vi "Window-Position control window.vi"() -> ()   [LabVIEW 2013]
uses:
  Program Files (x86)/National Instruments/LabVIEW 2013/user.lib/My Palettes.lib/Custom Controls/Directional Arrow Buttons/Arrow button-East.ctl
  Program Files (x86)/National Instruments/LabVIEW 2013/user.lib/My Palettes.lib/Custom Controls/Directional Arrow Buttons/Arrow button-West.ctl
  Program Files (x86)/National Instruments/LabVIEW 2013/user.lib/My Palettes.lib/Custom Controls/Directional Arrow Buttons/Arrow button-North.ctl
  Program Files (x86)/National Instruments/LabVIEW 2013/user.lib/My Palettes.lib/Custom Controls/Directional Arrow Buttons/Arrow button-South.ctl
  Program Files (x86)/National Instruments/LabVIEW 2013/user.lib/My Palettes.lib/Custom Controls/Directional Arrow Buttons/Arrow button-North west.ctl
  Program Files (x86)/National Instruments/LabVIEW 2013/user.lib/My Palettes.lib/Custom Controls/Directional Arrow Buttons/Arrow button-North east.ctl
  Program Files (x86)/National Instruments/LabVIEW 2013/user.lib/My Palettes.lib/Custom Controls/Directional Arrow Buttons/Arrow button-South west.ctl
  Program Files (x86)/National Instruments/LabVIEW 2013/user.lib/My Palettes.lib/Custom Controls/Directional Arrow Buttons/Arrow button-South east.ctl
  User Interface/Windows/Position control window/Typedefs/Pos Ctrl States.ctl
  User Interface/Windows/Position control window/Typedefs/Pos Ctrl queue data cluster.ctl
  User Interface/Windows/Position control window/Typedefs/Pos Ctrl window refs cluster.ctl
  Typedefs/Movement mode.ctl
  Peripherals Control/XYZ Stage/Typedefs/XYZ stage states.ctl
  Typedefs/Axis of movement.ctl
  User Interface/Windows/Position control window/Globals/Pos ctrl window globals.vi
  Global Variables/General Globals.vi
  Peripherals Control/XYZ Stage/Globals/gl_XYZStage globals.vi
  Typedefs/Save-Load enum.ctl
  Peripherals Control/XYZ Stage/Typedefs/XYZ channel ring.ctl
  Peripherals Control/XYZ Stage/Typedefs/XYZ stage data.ctl
panel:
  in  "Motor E-Stop":bool
  out "# elements in queue":i32
  out "x+1":dbl
  in  "Y Coordinate ctrl":sgl min=-20000 max=20000 step=0.1 format="Y:%#_g um"
  out "Close":bool
  in  "Z step (um)":sgl=1.0 min=0.1 max=1000 step=0.1 format="%#_6f"
  in  "Z Coordinate ctrl":sgl min=-20000 max=20000 step=0.1 format="Z:%#.1f um"
  in  "Z move down":T1
  in  "Z move up":T2
  out "Z-axis section":string
  in  "Step = size of image":bool
  in  "XY step (um)":sgl=1.0 min=0.1 max=10000 step=0.1
  out "State":T3
  out "Last button name":string
  out "Event loop":i32
  out "Elapsed Time (s)":dbl format="%#.1g"
  in  "Speed setting ctrl":i32=1000 min=1000 max=50000 step=1 format="Speed\n%#_6g\num/sec"
  in  "Speed down":bool
  in  "Speed up":bool
  in  "X Coordinate ctrl":sgl min=-20000 max=20000 step=0.1 format="X:%#_g um"
  in  "Down-right":T4
  in  "Down-left":T5
  in  "Up-right":T6
  in  "Up-left":T7
  in  "Down":T1
  in  "Up":T2
  in  "Left":T8
  in  "Right":T9
  # "Speed"
  # "X-Y Movement"
  # "Z Movement"
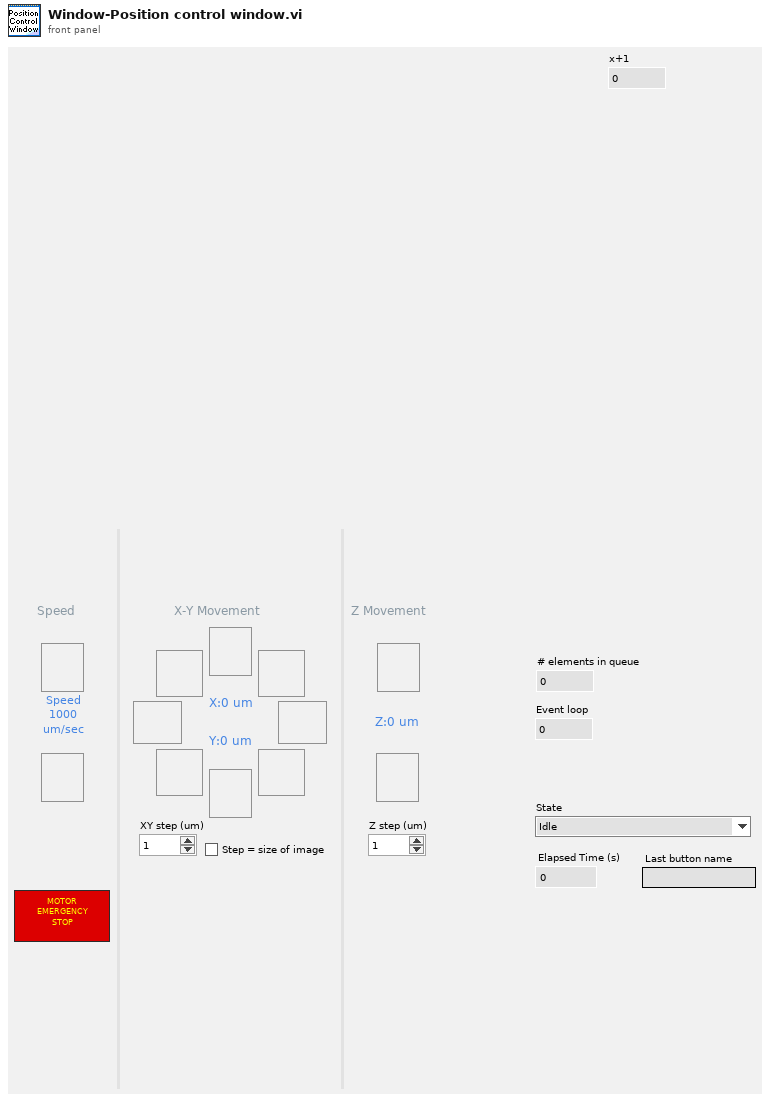
[diagram p1: front panel]
types:
  T1 = typedef "Arrow button-South.ctl" = bool
  T2 = typedef "Arrow button-North.ctl" = bool
  T3 = typedef "Pos Ctrl States.ctl" = enum16{"Idle", "Count-down", "Request single step (ack.)", "Request single step (no ack.)", "Request continuous movement", "Request movement stop"}
  T4 = typedef "Arrow button-South east.ctl" = bool
  T5 = typedef "Arrow button-South west.ctl" = bool
  T6 = typedef "Arrow button-North east.ctl" = bool
  T7 = typedef "Arrow button-North west.ctl" = bool
  T8 = typedef "Arrow button-West.ctl" = bool
  T9 = typedef "Arrow button-East.ctl" = bool
  T10 = typedef "Pos Ctrl window refs cluster.ctl" = cluster{"menu reference":refnum<k9>, "X Coordinate ctrl":refnum<vi>, "Y Coordinate ctrl":refnum<vi>, "Z Coordinate ctrl":refnum<vi>, "Speed setting ctrl":refnum<vi>, "Up":refnum<vi>, "Down":refnum<vi>, "Left":refnum<vi>, "Right":refnum<vi>, "Z move up":refnum<vi>, "Z move down":refnum<vi>, "Down-left":refnum<vi>, "Down-right":refnum<vi>, "Up-left":refnum<vi>, "Up-right":refnum<vi>, "Step = size of image":refnum<vi>, "XY step (um)":refnum<vi>, "Z step (um)":refnum<vi>}
  T11 = typedef "Pos Ctrl queue data cluster.ctl" = cluster{"State":T3, "variant":variant}
  T12 = enum32{"Invalid", "Standard", "Closed", "Hidden", "Minimized", "Maximized"}
  T13 = typedef "XYZ stage states.ctl" = enum16{"Dequeue", "Initialize", "Read Position", "Read Speed Setting", "Move", "Set Max Speed", "Reset Axis", "Stop all movement"}
  T14 = typedef "Axis of movement.ctl" = enum16{"None", "X-axis", "Y-Axis", "-45 deg Axis", "+45 deg Axis", "Z-Axis"}
  T15 = enum8{"Enabled", "Disabled", "Disabled and Grayed Out"}
  T16 = typedef "XYZ stage data.ctl" = cluster{"Command":T13, "Channel":T17, "X":sgl, "Y":sgl, "Z":sgl, "Speed":i32, "Zero":bool, "Use acknowledgement?":bool}
  T17 = typedef "XYZ channel ring.ctl" = string
  T18 = typedef "Save-Load enum.ctl" = enum16{"Save to file", "Load from file", "Compare from file"}
  T19 = typedef "Movement mode.ctl" = enum16{"Move the frame", "Move the feature"}
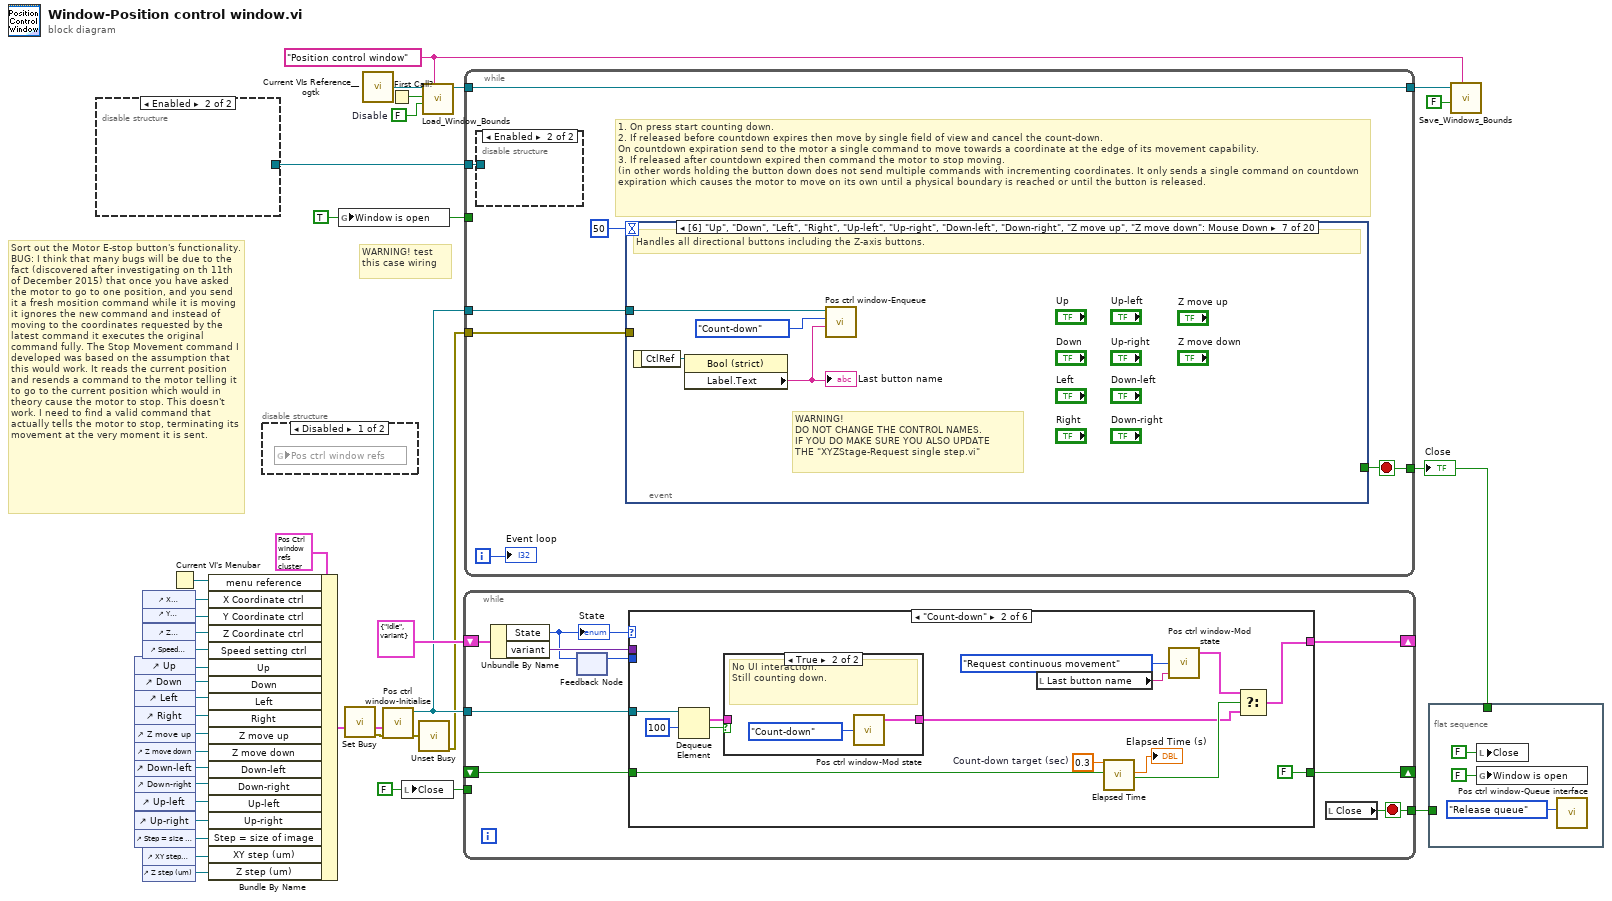
[diagram p0: block diagram]
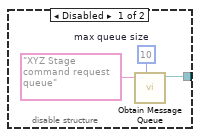
[diagram p2: hidden frame]
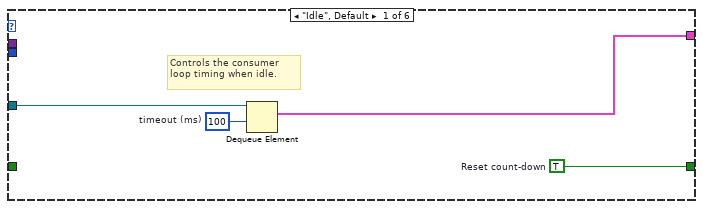
[diagram p4: hidden frame]
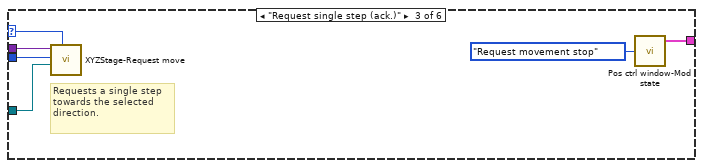
[diagram p6: hidden frame]
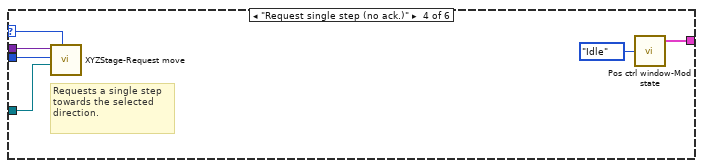
[diagram p7: hidden frame]
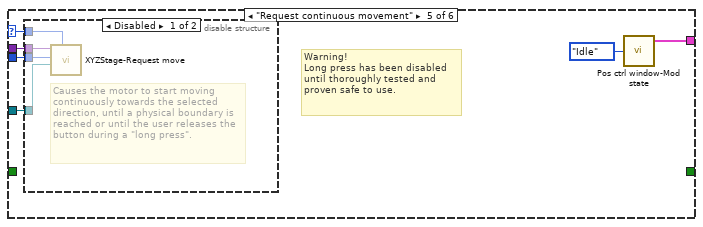
[diagram p8: hidden frame]
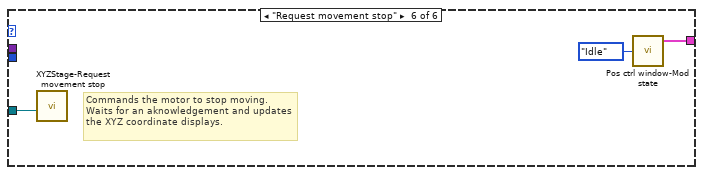
[diagram p10: hidden frame]
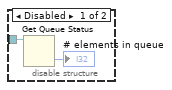
[diagram p11: hidden frame]
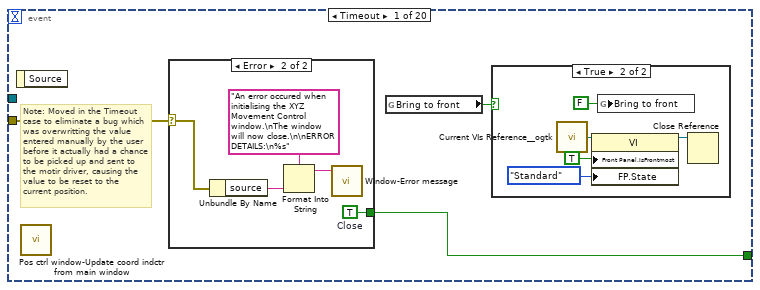
[diagram p12: hidden frame]
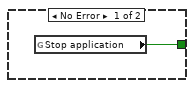
[diagram p14: hidden frame]
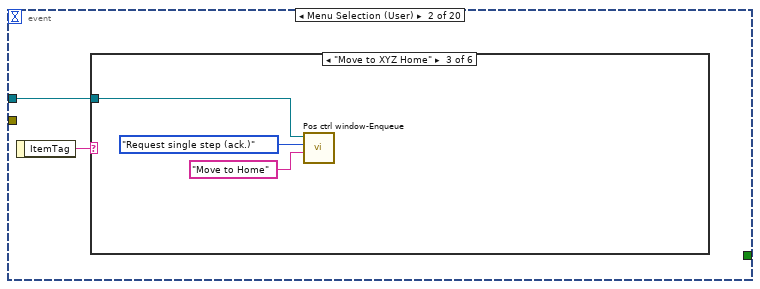
[diagram p15: hidden frame]
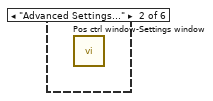
[diagram p17: hidden frame]
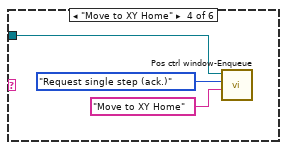
[diagram p18: hidden frame]
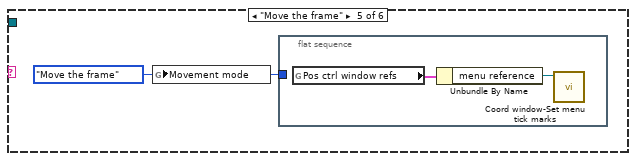
[diagram p19: hidden frame]
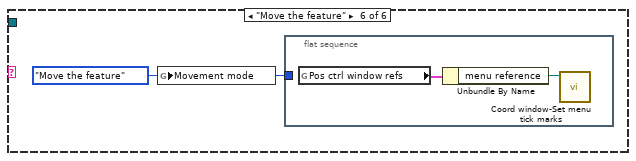
[diagram p20: hidden frame]
diagram:
  w10 = FALSE  # Disable
  w8 = "Position control window" ("Window Name (i.e. Key)")
  w14 = TRUE ("Bring to front")
  w25 = FALSE ("Close")
  # "Sort out the Motor E-stop button's functionality.\nBUG: I think that many bugs will be due to the fact (discovered after investigating on th 11th of December 2015) that once you have asked the motor to go to one position, and you send it a fresh mosition command while it is moving it ignores the new command and instead of moving to the coordinates requested by the latest command it executes the original command fully. The Stop Movement command I developed was based on the assumption that this would work. It reads the current position and resends a command to the motor telling it to go to the current position which would in theory cause the motor to stop. This doesn't work. I need to find a valid command that actually tells the motor to stop, terminating its movement at the very moment it is sent."
  # "WARNING! test this case wiring"
  n1 = disable-structure shown="Enabled" {
    disable-tunnel: [w38 _] -> w6
    frame Disabled {
      w40 = 10  # max queue size
      n2 = call "Obtain Message Queue.vi"("max queue size (-1, unlimited)"=w40, "Queue name"="XYZ Stage command request queue") -> ("Message Queue"=w38:refnum<queue>)  [unwired: 8 in, 1 out]
    }
    frame Enabled {
    }
  }
  n3 = control-ref of="Up"() -> (w35:refnum<vi>)
  n4 = control-ref of="Down"() -> (w34:refnum<vi>)
  n5 = control-ref of="Left"() -> (w33:refnum<vi>)
  n6 = control-ref of="Right"() -> (w32:refnum<vi>)
  n7 = control-ref of="Z move up"() -> (w31:refnum<vi>)
  n8 = control-ref of="Z move down"() -> (w30:refnum<vi>)
  n9 = control-ref of="Down-left"() -> (w29:refnum<vi>)
  n10 = control-ref of="Down-right"() -> (w28:refnum<vi>)
  n11 = control-ref of="Up-left"() -> (w27:refnum<vi>)
  n12 = control-ref of="Up-right"() -> (w26:refnum<vi>)
  n13 = control-ref of="Step = size of image"() -> (w23:refnum<vi>)
  n14 = control-ref of="X Coordinate ctrl"() -> (w18:refnum<vi>)
  n15 = control-ref of="Y Coordinate ctrl"() -> (w17:refnum<vi>)
  n16 = control-ref of="Z Coordinate ctrl"() -> (w16:refnum<vi>)
  n17 = control-ref of="Speed setting ctrl"() -> (w15:refnum<vi>)
  n18 = control-ref of="XY step (um)"() -> (w22:refnum<vi>)
  n19 = control-ref of="Z step (um)"() -> (w21:refnum<vi>)
  n20 = Current VI's Menubar() -> (w5:refnum<k9>)
  n21 = Bundle By Name(cluster=T10 {"menu reference"=refnum, "X Coordinate ctrl"=refnum, "Y Coordinate ctrl"=refnum, "Z Coordinate ctrl"=refnum, "Speed setting ctrl"=refnum, "Up"=refnum, "Down"=refnum, "Left"=refnum, "Right"=refnum, "Z move up"=refnum, "Z move down"=refnum, "Down-left"=refnum, "Down-right"=refnum, "Up-left"=refnum, "Up-right"=refnum, "Step = size of image"=refnum, "XY step (um)"=refnum, "Z step (um)"=refnum} ("Pos ctrl window refs"), "menu reference"=w5, "X Coordinate ctrl"=w18, "Y Coordinate ctrl"=w17, "Z Coordinate ctrl"=w16, "Speed setting ctrl"=w15, "Up"=w35, "Down"=w34, "Left"=w33, "Right"=w32, "Z move up"=w31, "Z move down"=w30, "Down-left"=w29, "Down-right"=w28, "Up-left"=w27, "Up-right"=w26, "Step = size of image"=w23, "XY step (um)"=w22, "Z step (um)"=w21) -> (w19:T10)
  n22 = disable-structure shown="Disabled" {
    frame Disabled {
      n23 = global read "Pos ctrl window globals.vi" "Pos ctrl window refs"() -> ()  [unwired: 1 in]
    }
    frame Enabled {
    }
  }
  n24 = global write "Pos ctrl window globals.vi" "Window is open"(w14) -> ()
  n25 = call <vilib>:"Set Busy.vi"() -> ("error out"=w3:errorcluster)  [unwired: 10 in, 1 out]
  n26 = call "Current VIs Reference__ogtk.vi"() -> ("Current VI's reference"=w13:refnum<vi>)  [unwired: 5 in]
  n27 = call "Pos ctrl window-Initialise.vi"("error in (no error)"=w3, "Pos ctrl window refs"=w19) -> ("error out"=w2:errorcluster, "XYZ movement ctrl window queue ref"=w20:refnum<queue>)  [unwired: 8 in]
  n28 = First Call?() -> (First Call?: T/F=w11:bool)
  n29 = local write "Close"(w25) -> ()
  n30 = call <vilib>:"Unset Busy.vi"("error in (no error)"=w2) -> ("error out"=w1:errorcluster)  [unwired: 10 in]
  n31 = call "Load_Window_Bounds.vi"("Window Name (i.e. Key)"=w8, "Disable"=w10, "First Call"=w11, "Window VI's Ref"=w13) -> ("reference out"=w12:refnum<vi>)  [unwired: 4 in, 3 out]
  n32 = while {
    tunnel: w20 -> [w49]
    shift-right: [w48] -> _
    shift-left: T11 {"State"=enum."Idle", "variant"=variant} ("Pos Ctrl queue data cluster") -> [w45]
    shift-right: [w47] -> _
    shift-left: _ -> [w46]
    tunnel: w25 -> [_]
    tunnel: [w41] -> w24
    stop <- w41 stop-if-true
    n33 = Unbundle By Name(w45) -> ("State"=w43:T3, "variant"=w44:variant)
    "State" <- w43
    n34 = feedback-in #1(w43) -> ()
    n35 = feedback #1() -> (w42:T3)  [unwired: 1 in]
    n36 = case shown="\"Count-down\"" w43 {
      selector: w43 -> [_ _ w71 w77 w83 _]
      tunnel: w49 -> [w52 w66 w73 w79 w86 w93]
      tunnel: [w50 w55 w75 w81 w87 w94] -> w48
      tunnel: [w51 FALSE _ _ _ _] -> w47
      tunnel: w46 -> [_ w63 _ _ _ _]
      tunnel: w44 -> [_ _ w74 w80 w85 _]
      tunnel: w42 -> [_ _ w72 w78 w84 _]
      frame "Idle", Default {
        w51 = TRUE  # Reset count-down
        w53 = 100  # timeout (ms)
        # "Controls the consumer loop timing when idle."
        n37 = Dequeue Element(queue=w52, timeout in ms (-1)=w53) -> (element=w50:T11)  [unwired: 1 in, 3 out]
      }
      frame "Count-down" {
        w64 = 0.3  # Count-down target (sec)
        n38 = Dequeue Element(queue=w66, timeout in ms (-1)=100) -> (element=w61:T11, timed out?=w62:bool)  [unwired: 1 in, 2 out]
        n39 = case shown="True" w62 {
          tunnel: [w68 w69] -> w56
          tunnel: w61 -> [w68 _]
          frame False {
            # "Queue element received.\nUI interaction detected."
          }
          frame True {
            # "No UI interaction.\nStill counting down."
            n40 = call "Pos ctrl window-Mod state.vi"("States"=Pos_Ctrl_States."Count-down") -> ("Modified queue element"=w69:T11)  [unwired: 4 in]
          }
        }
        n41 = local read "Last button name"() -> (w54:string)
        n42 = call "Elapsed Time"("Time Target (s)"=w64, "Reset"=w63) -> ("Elapsed Time (s)"=→"Elapsed Time (s)":dbl, "Time has Elapsed"=w57:bool)  [unwired: 10 in, 6 out]
        n43 = call "Pos ctrl window-Mod state.vi"("variant"=w54, "States"=Pos_Ctrl_States."Request continuous movement") -> ("Modified queue element"=w59:T11)  [unwired: 3 in]
        n44 = Select(t=w59, s=w57, f=w56) -> (s? t:f=w55:T11)
      }
      frame "Request single step (ack.)" {
        # "Requests a single step towards the selected direction."
        n45 = call "XYZStage-Request move.vi"("Current State"=w71, "Pos ctrl window queue"=w73, "Previous State"=w72, "variant"=w74) -> ()  [unwired: 8 in]
        n46 = call "Pos ctrl window-Mod state.vi"("States"=Pos_Ctrl_States."Request movement stop") -> ("Modified queue element"=w75:T11)  [unwired: 4 in]
      }
      frame "Request single step (no ack.)" {
        # "Requests a single step towards the selected direction."
        n47 = call "XYZStage-Request move.vi"("Current State"=w77, "Pos ctrl window queue"=w79, "Previous State"=w78, "variant"=w80) -> ()  [unwired: 8 in]
        n48 = call "Pos ctrl window-Mod state.vi"("States"=Pos_Ctrl_States."Idle") -> ("Modified queue element"=w81:T11)  [unwired: 4 in]
      }
      frame "Request continuous movement" {
        # "Warning!\nLong press has been disabled until thoroughly tested and proven safe to use."
        n49 = disable-structure shown="Disabled" {
          disable-tunnel: w86 -> [w92 _]
          disable-tunnel: w85 -> [w91 _]
          disable-tunnel: w84 -> [w90 _]
          disable-tunnel: w83 -> [w89 _]
          frame Disabled {
            # "Causes the motor to start moving continuously towards the selected direction, until a physical boundary is reached or until the user releases the button during a \"long press\"."
            n50 = call "XYZStage-Request move.vi"("Current State"=w89, "Pos ctrl window queue"=w92, "Previous State"=w90, "variant"=w91) -> ()  [unwired: 8 in]
          }
          frame Enabled {
          }
        }
        n51 = call "Pos ctrl window-Mod state.vi"("States"=Pos_Ctrl_States."Idle") -> ("Modified queue element"=w87:T11)  [unwired: 4 in]
      }
      frame "Request movement stop" {
        # "Commands the motor to stop moving.\nWaits for an aknowledgement and updates the XYZ coordinate displays."
        n52 = call "XYZStage-Request movement stop.vi"("Pos ctrl window queue"=w93) -> ()  [unwired: 11 in]
        n53 = call "Pos ctrl window-Mod state.vi"("States"=Pos_Ctrl_States."Idle") -> ("Modified queue element"=w94:T11)  [unwired: 4 in]
      }
    }
    n54 = local read "Close"() -> (w41:bool)
  }
  n55 = while {
    tunnel: w20 -> [w101]
    tunnel: [w99] -> w4
    tunnel: w1 -> [w98]
    tunnel: w14 -> [_]
    tunnel: w12 -> [w97]
    tunnel: [w97] -> w9
    tunnel: w6 -> [w96]
    i -> [w100]
    stop <- w99 stop-if-true
    # "1. On press start counting down.\n2. If released before countdown expires then move by single field of view and cancel the count-down.\nOn countdown expiration send to the motor a single command to move towards a coordinate at the edge of its movement capability.\n3. If released after countdown expired then command the motor to stop moving.\n(in other words holding the button down does not send multiple commands with incrementing coordinates. It only sends a single command on countdown expiration which causes the motor to move on its own until a physical boundary is reached or until the button is released."
    n56 = disable-structure shown="Enabled" {
      disable-tunnel: w96 -> [w104 _]
      frame Disabled {
        n57 = Get Queue Status(queue=w104) -> (# elements in queue=→"# elements in queue":i32)  [unwired: 2 in, 7 out]
      }
      frame Enabled {
      }
    }
    n58 = event shown="[6] \"Up\", \"Down\", \"Left\", \"Right\", \"Up-left\", \"Up-right\", \"Down-left\", \"Down-right\", \"Z move up\", \"Z move down\": Mouse Down" {
      selector: _ -> [_ _ _ _ _ _ _ _ _ _ _ _ _ _ _ _ _ _ _ _]
      dyn-events: _ -> [_ _ _ _ _ _ _ _ _ _ _ _ _ _ _ _ _ _ _ _]
      timeout: 50 -> [_ _ _ _ _ _ _ _ _ _ _ _ _ _ _ _ _ _ _ _]
      tunnel: w101 -> [_ w119 w136 _ _ _ w172 w175 w183 _ _ _ _ _ _ _ _ _ w199 _]
      tunnel: [w106 _ _ _ _ _ _ _ _ _ _ _ _ _ _ _ _ _ _ TRUE] -> w99
      tunnel: w98 -> [w107 _ _ _ _ _ _ _ _ _ _ _ _ _ _ _ _ _ _ _]
      event Timeout {
        # "Note: Moved in the Timeout case to eliminate a bug which was overwritting the value entered manually by the user before it actually had a chance to be picked up and sent to the motir driver, causing the value to be reset to the current position."
        n59 = event-data() -> ()  [unwired: 1 in, 1 out]
        n60 = call "Pos ctrl window-Update coord indctr from main window.vi"() -> ()  [unwired: 12 in]
        n61 = case shown="Error" w107 {
          selector: w107 -> [_ w115]
          tunnel: [w113 w118] -> w106
          frame No Error {
            n62 = global read "General Globals.vi" "Stop application"() -> (w113:bool)
          }
          frame Error {
            w118 = TRUE  # Close
            n63 = Unbundle By Name(w115) -> ("source"=w114:string)
            n64 = Format Into String(format string="An error occured when initialising the XYZ Movement Control window.\nThe window will now close.\n\nERROR DETAILS:\n%s" ("Error Source"), w114) -> (resulting string=w117:string)  [unwired: 2 in, 1 out]
            n65 = call "Window-Error message.vi"("Message"=w117) -> ()  [unwired: 10 in, 1 out]
          }
        }
        n66 = global read "Pos ctrl window globals.vi" "Bring to front"() -> (w105:bool)
        n67 = case shown="True" w105 {
          frame False {
          }
          frame True {
            n68 = call "Current VIs Reference__ogtk.vi"() -> ("Current VI's reference"=w111:refnum<vi>)  [unwired: 5 in]
            n69 = property class="VI"(reference=w111, "Front Panel.IsFrontmost"=TRUE ("Front Panel Window:Is Frontmost"), "FP.State"=T12."Standard" ("Front Panel Window:State")) -> (reference out=w110:refnum<vi>)  [unwired: 1 in, 1 out]
            n70 = global write "Pos ctrl window globals.vi" "Bring to front"(FALSE ("Bring to front")) -> ()
            n71 = Close Reference(reference=w110) -> ()  [unwired: 1 in, 1 out]
          }
        }
      }
      event Menu Selection (User) {
        n72 = event-data() -> ("ItemTag"=w120:string)  [unwired: 1 in]
        n73 = case shown="\"Move to XYZ Home\"" w120 {
          tunnel: w119 -> [_ _ w121 w124 _ _]
          frame Default {
          }
          frame "Advanced Settings..." {
            n74 = call "Pos ctrl window-Settings window.vi"() -> ()  [unwired: 11 in, 1 out]
          }
          frame "Move to XYZ Home" {
            n75 = call "Pos ctrl window-Enqueue.vi"("variant"="Move to Home" ("Last button name"), "States"=Pos_Ctrl_States."Request single step (ack.)", "Pos ctrl window queue"=w121) -> ()  [unwired: 8 in, 1 out]
          }
          frame "Move to XY Home" {
            n76 = call "Pos ctrl window-Enqueue.vi"("variant"="Move to XY Home" ("Last button name"), "States"=Pos_Ctrl_States."Request single step (ack.)", "Pos ctrl window queue"=w124) -> ()  [unwired: 8 in, 1 out]
          }
          frame "Move the frame" {
            w127 = Movement_mode."Move the frame" ("Movement mode")
            n77 = global write "Pos ctrl window globals.vi" "Movement mode"(w127) -> ()
            n78 = flat-sequence {
              tunnel: w127 -> [_]
              frame #0 {
                n79 = global read "Pos ctrl window globals.vi" "Pos ctrl window refs"() -> (w128:T10)
                n80 = Unbundle By Name(w128) -> ("menu reference"=w129:refnum<k9>)
                n81 = call "Coord window-Set menu tick marks.vi"("Menu in"=w129) -> ()  [unwired: 9 in, 2 out]
              }
            }
          }
          frame "Move the feature" {
            w130 = Movement_mode."Move the feature" ("Movement mode")
            n82 = global write "Pos ctrl window globals.vi" "Movement mode"(w130) -> ()
            n83 = flat-sequence {
              tunnel: w130 -> [_]
              frame #0 {
                n84 = global read "Pos ctrl window globals.vi" "Pos ctrl window refs"() -> (w131:T10)
                n85 = Unbundle By Name(w131) -> ("menu reference"=w132:refnum<k9>)
                n86 = call "Coord window-Set menu tick marks.vi"("Menu in"=w132) -> ()  [unwired: 9 in, 2 out]
              }
            }
          }
        }
      }
      event Mouse Wheel {
        # "Controls the stage when scrolling the mouse wheel over the Up or Down arrow key."
        n87 = event-data() -> ("Delta"=w135:i32)  [unwired: 1 in]
        n88 = global read "Pos ctrl window globals.vi" "Axis of movement"() -> (w133:T14)
        n89 = Greater Than 0?(x=w135) -> (x > 0?=w134:bool)
        n90 = case shown="Default" w133 {
          selector: w133 -> [_ w137]
          tunnel: w136 -> [_ w143]
          tunnel: w134 -> [_ w141]
          frame "None" {
          }
          frame Default {
            n91 = case shown="\"Z-Axis\"" w137 {
              tunnel: [w145 w149 w153 w158 w162] -> w142
              tunnel: w141 -> [w146 w150 w154 w157 w161]
              frame "X-axis", Default {
                n92 = case shown="True" w146 {
                  tunnel: ["Left" "Right"] -> w145
                  frame False {
                    # "Reducing X"
                  }
                  frame True {
                    # "Increasing X"
                  }
                }
              }
              frame "-45 deg Axis" {
                n93 = case shown="True" w150 {
                  tunnel: ["Down-right" "Up-left"] -> w149
                  frame False {
                  }
                  frame True {
                  }
                }
              }
              frame "+45 deg Axis" {
                n94 = case shown="True" w154 {
                  tunnel: ["Down-left" "Up-right"] -> w153
                  frame False {
                  }
                  frame True {
                  }
                }
              }
              frame "Y-Axis" {
                n95 = case shown="True" w157 {
                  tunnel: ["Down" "Up"] -> w158
                  frame False {
                    # "Reducing Y"
                  }
                  frame True {
                    # "Increasing Y"
                  }
                }
              }
              frame "Z-Axis" {
                n96 = case shown="False" w161 {
                  tunnel: ["Z move down" "Z move up"] -> w162
                  frame False {
                    # "Reducing Z"
                  }
                  frame True {
                    # "Increasing Z"
                  }
                }
              }
            }
            n97 = local write "Last button name"(w142) -> ()
            n98 = feedback #2(0.0) -> (w140:dbl)
            n99 = Increment(x=w140) -> (x+1=w139:dbl)
            "x+1" <- w139
            n100 = feedback-in #2(w139) -> ()
            n101 = call "Pos ctrl window-Enqueue.vi"("variant"=w142, "States"=Pos_Ctrl_States."Request single step (no ack.)", "Pos ctrl window queue"=w143) -> ()  [unwired: 8 in, 1 out]
          }
        }
      }
      event "Speed setting ctrl": Value Change {
        n102 = event-data() -> ("NewVal"=w165:i32)  [unwired: 1 in]
        n103 = call "XYZStage-Request speed setting command.vi"("Speed to set"=w165, "Which speed setting command?"=XYZ_stage_states."Set Max Speed" ("Command")) -> ()  [unwired: 9 in, 1 out]
      }
      event "Speed up": Value Change {
        n104 = event-data() -> ()  [unwired: 1 in, 1 out]
        n105 = call "XYZStage-Increase or reduce speed setting.vi"("Function"=enum16{"Increase speed", "Reduce speed"}."Increase speed") -> ()  [unwired: 11 in]
      }
      event "Speed down": Value Change {
        n106 = event-data() -> ()  [unwired: 1 in, 1 out]
        n107 = call "XYZStage-Increase or reduce speed setting.vi"("Function"=enum16{"Increase speed", "Reduce speed"}."Reduce speed") -> ()  [unwired: 11 in]
      }
      event Mouse Down {
        # "WARNING!\nDO NOT CHANGE THE CONTROL NAMES.\nIF YOU DO MAKE SURE YOU ALSO UPDATE\nTHE \"XYZStage-Request single step.vi\""
        # "Handles all directional buttons including the Z-axis buttons."
        n108 = event-data() -> ("CtlRef"=w170:refnum<vi>)  [unwired: 1 in]
        n109 = property class="Bool (strict)"(reference=w170) -> ("Label.Text"=w169:string)  [unwired: 1 in, 2 out]
        "Last button name" <- w169
        n110 = call "Pos ctrl window-Enqueue.vi"("variant"=w169, "States"=Pos_Ctrl_States."Count-down", "Pos ctrl window queue"=w172) -> ()  [unwired: 8 in, 1 out]
      }
      event "Z Coordinate ctrl", "X Coordinate ctrl", "Y Coordinate ctrl": Value Change {
        n111 = event-data() -> ("CtlRef"=w174:refnum<vi>)  [unwired: 1 in]
        n112 = property class="DigNum (strict)"(reference=w174) -> ("Label.Text"=w173:string)  [unwired: 1 in, 2 out]
        n113 = local write "Last button name"(w173) -> ()
        n114 = call "Pos ctrl window-Enqueue.vi"("variant"=w173, "States"=Pos_Ctrl_States."Request single step (ack.)", "Pos ctrl window queue"=w175) -> ()  [unwired: 8 in, 1 out]
      }
      event Mouse Up {
        # "Also bundles the name of the control.\nThis is then used to determine the direction.\nHandles all the directional buttons."
        # "Handles all directional buttons including the Z-axis buttons."
        n115 = event-data() -> ("CtlRef"=w182:refnum<vi>)  [unwired: 1 in]
        n116 = local read "State"() -> (w180:T3)
        n117 = Equal?(x=Pos_Ctrl_States."Count-down", y=w180) -> (x = y?=w178:bool)
        n118 = case shown="True" w178 {
          tunnel: [Pos_Ctrl_States."Request movement stop" ("States") Pos_Ctrl_States."Request single step (ack.)" ("States")] -> w177
          frame False {
            # "Long-press count down has completed"
          }
          frame True {
            # "Still in count-down for long-press"
          }
        }
        n119 = property class="Bool (strict)"(reference=w182) -> ("Label.Text"=w181:string)  [unwired: 1 in, 2 out]
        n120 = local write "Last button name"(w181) -> ()
        n121 = call "Pos ctrl window-Enqueue.vi"("variant"=w181, "States"=w177, "Pos ctrl window queue"=w183) -> ()  [unwired: 8 in, 1 out]
      }
      event "Y Coordinate ctrl": Mouse Enter {
        n122 = event-data() -> ()  [unwired: 1 in, 1 out]
        n123 = global write "Pos ctrl window globals.vi" "Axis of movement"(Axis_of_movement."Y-Axis" ("Axis of movement")) -> ()
      }
      event "X Coordinate ctrl": Mouse Enter {
        n124 = event-data() -> ()  [unwired: 1 in, 1 out]
        n125 = global write "Pos ctrl window globals.vi" "Axis of movement"(Axis_of_movement."X-axis" ("Axis of movement")) -> ()
      }
      event Mouse Enter {
        n126 = event-data() -> ()  [unwired: 1 in, 1 out]
        n127 = global write "Pos ctrl window globals.vi" "Axis of movement"(Axis_of_movement."-45 deg Axis" ("Axis of movement")) -> ()
      }
      event Mouse Enter {
        n128 = event-data() -> ()  [unwired: 1 in, 1 out]
        n129 = global write "Pos ctrl window globals.vi" "Axis of movement"(Axis_of_movement."+45 deg Axis" ("Axis of movement")) -> ()
      }
      event "Z-axis section": Mouse Enter {
        # "This indicator is hidden and causes the Z-slider to come in focus on a \"mouse enter\" event."
        n130 = event-data() -> ()  [unwired: 1 in, 1 out]
        n131 = global write "Pos ctrl window globals.vi" "Axis of movement"(Axis_of_movement."Z-Axis" ("Axis of movement")) -> ()
      }
      event "Speed up", "Speed down", "Z-axis section", "X Coordinate ctrl", "Y Coordinate ctrl": Mouse Leave {
        n132 = event-data() -> ()  [unwired: 1 in, 1 out]
        n133 = global write "Pos ctrl window globals.vi" "Axis of movement"(Axis_of_movement."None" ("Axis of movement")) -> ()
      }
      event "XY step (um)": Value Change {
        n134 = event-data() -> ()  [unwired: 1 in, 1 out]
        n135 = global write "Pos ctrl window globals.vi" "XY step (um)"("XY step (um)") -> ()
      }
      event "Z step (um)": Value Change {
        n136 = event-data() -> ()  [unwired: 1 in, 1 out]
        n137 = global write "Pos ctrl window globals.vi" "Z step (um)"("Z step (um)") -> ()
      }
      event "Step = size of image": Value Change {
        n138 = event-data() -> ()  [unwired: 1 in, 1 out]
        n139 = global write "Pos ctrl window globals.vi" "Step = size of image"("Step = size of image") -> ()
        n140 = Select(t=T15."Disabled and Grayed Out" ("Disabled"), s="Step = size of image", f=T15."Enabled" ("Disabled")) -> (s? t:f=w196:T15)
        n141 = property on="XY step (um)" class="DigNum (strict)"("DisabledEnum"=w196) -> ()  [unwired: 2 in, 2 out]
      }
      event "Motor E-Stop": Value Change {
        n142 = event-data() -> ()  [unwired: 1 in, 1 out]
        n143 = Flush Queue(queue=w199) -> (error out=w198:errorcluster)  [unwired: 1 in, 2 out]
        n144 = flat-sequence {
          tunnel: w198 -> [_]
          frame #0 {
            n145 = disable-structure shown="Enabled" {
              frame Disabled {
                n146 = Bundle By Name(cluster=T16 {"Command"=enum."Initialize", "Channel"="Z", "X"=0.0, "Y"=0.0, "Z"=0.0, "Speed"=0, "Zero"=FALSE, "Use acknowledgement?"=FALSE} ("XYZ Stage data to queue"), "Use acknowledgement?"=FALSE) -> (w203:T16)
                n147 = call "XYZ Stage-Command request module.vi"("Command"=XYZ_stage_states."Stop all movement", "XYZ Stage data to queue"=w203) -> ()  [unwired: 5 in, 5 out]
              }
              frame Enabled {
                n148 = global write "gl_XYZStage globals.vi" "Motor E-stop"(TRUE ("Motor E-stop")) -> ()
              }
            }
          }
        }
      }
      event Panel Close {
        # "The XYZ window setup is now saved as part of the user-profile save functionality and no longer auto-saved when the window is closed."
        n149 = event-data() -> ()  [unwired: 1 in, 1 out]
        n150 = disable-structure shown="Disabled" {
          frame Disabled {
            n151 = call "Read-Write XYZ movement setup.vi"("Function"=Save-Load_enum."Save to file") -> ()  [unwired: 10 in, 1 out]
          }
          frame Enabled {
          }
        }
      }
    }
    "Event loop" <- w100
  }
  "Close" <- w4
  n152 = flat-sequence {
    tunnel: w24 -> [_]
    tunnel: w4 -> [_]
    frame #0 {
      n153 = local write "Close"(FALSE ("Close")) -> ()
      n154 = global write "Pos ctrl window globals.vi" "Window is open"(FALSE ("Bring to front")) -> ()
      n155 = call "Pos ctrl window-Queue interface.vi"("Function"=enum16{"None", "Release queue"}."Release queue") -> ()  [unwired: 9 in, 2 out]
    }
  }
  n156 = call "Save_Windows_Bounds.vi"("Window Name (i.e. Key)"=w8, "Front Panel Window:Open"=FALSE, "Window VI's Ref"=w9) -> ()  [unwired: 8 in, 1 out]
